vi "15_NOV_UPDATE.vi"() -> ()   [LabVIEW 2020]
uses:
  <vilib>/Utility/file.llb/Write Delimited Spreadsheet (DBL).vi
  <instrlib>/Agilent B2900 Series/Agilent B2900 Series.lvlib
panel:
  in  "Save Data":bool
  out "Y -axis":string
  out "X -axis":string
  out "String":string
  out "SCPI Command":string
  out "?":bool
  in  "Time interval between iterations (seconds)":dbl
  out "?":cluster{"X":dbl[], "Y":dbl[]}[](graph)
  out "Waveform Chart":dbl(graph)
  out "Measured Output Value":dbl
  in  "SELECT DEVICE":refnum<visa-resource-name>="USB0::0x0957::0x8E18::MY51140695::INSTR"
  out "Resolution":dbl format="%#_6f"
  out "Instantaneous Input Value":dbl format="%#_6f"
  in  "Final Value":dbl
  in  "Initial Value":dbl
  in  "Steps":dbl
  in  "Measure (OUTPUT)":enum16{"Voltage", "Current"}(ring)
  in  "Source":enum16{"Voltage", "Current"}(ring)
  in  "Channel":u16(ring) items=["1", "2"]
  # "(INPUT)"
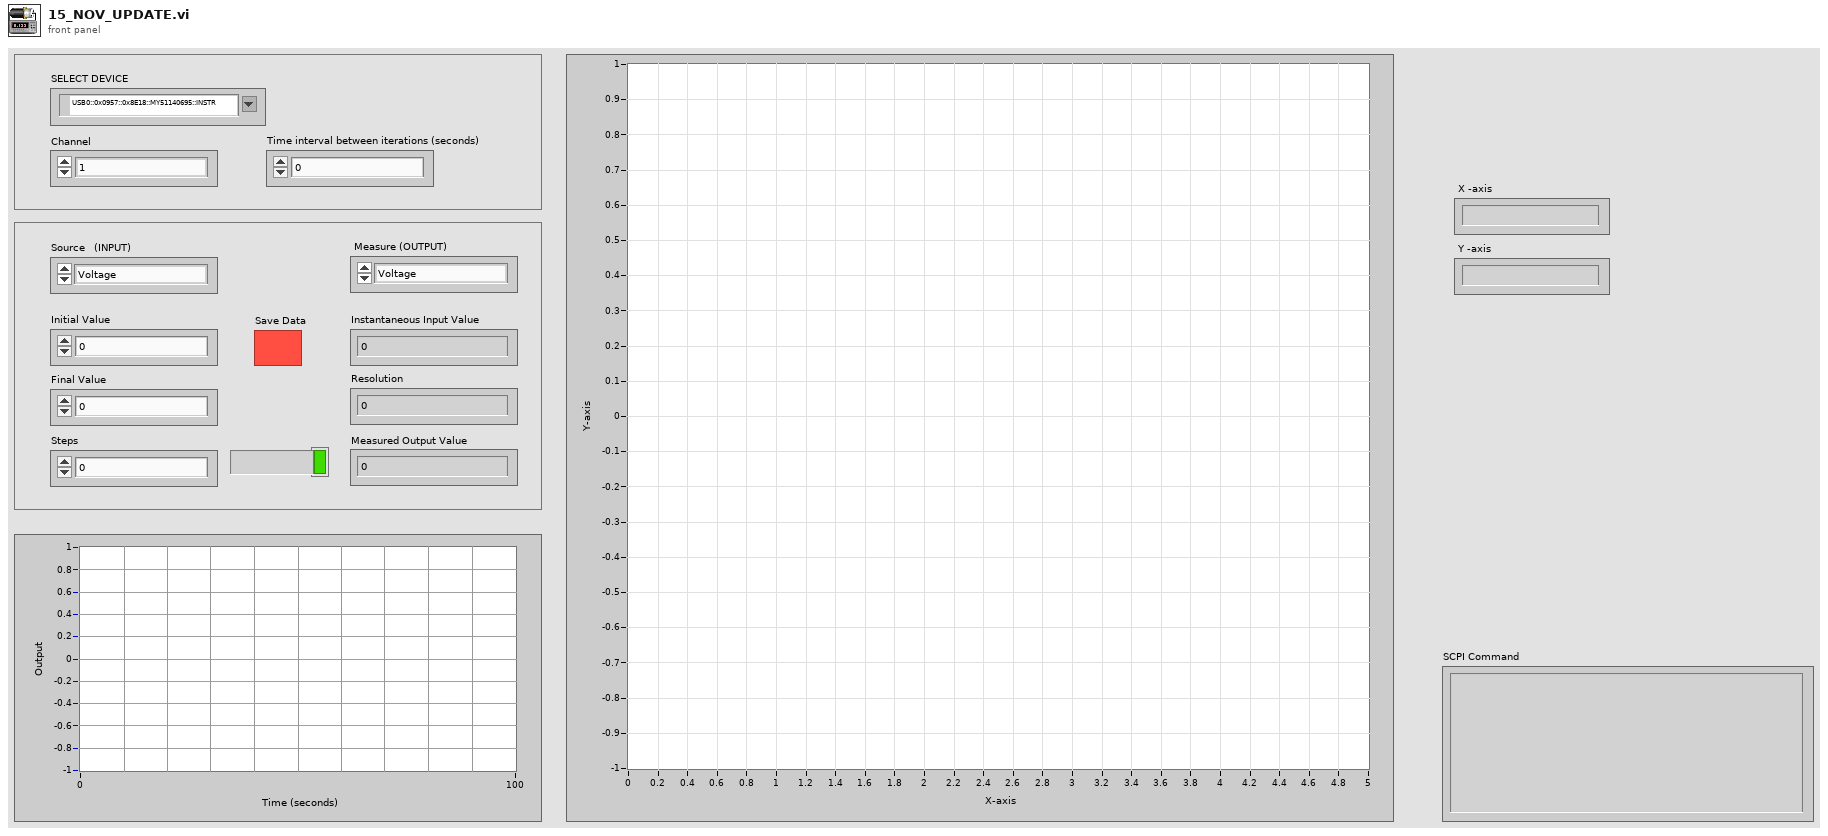
[diagram p1: front panel]
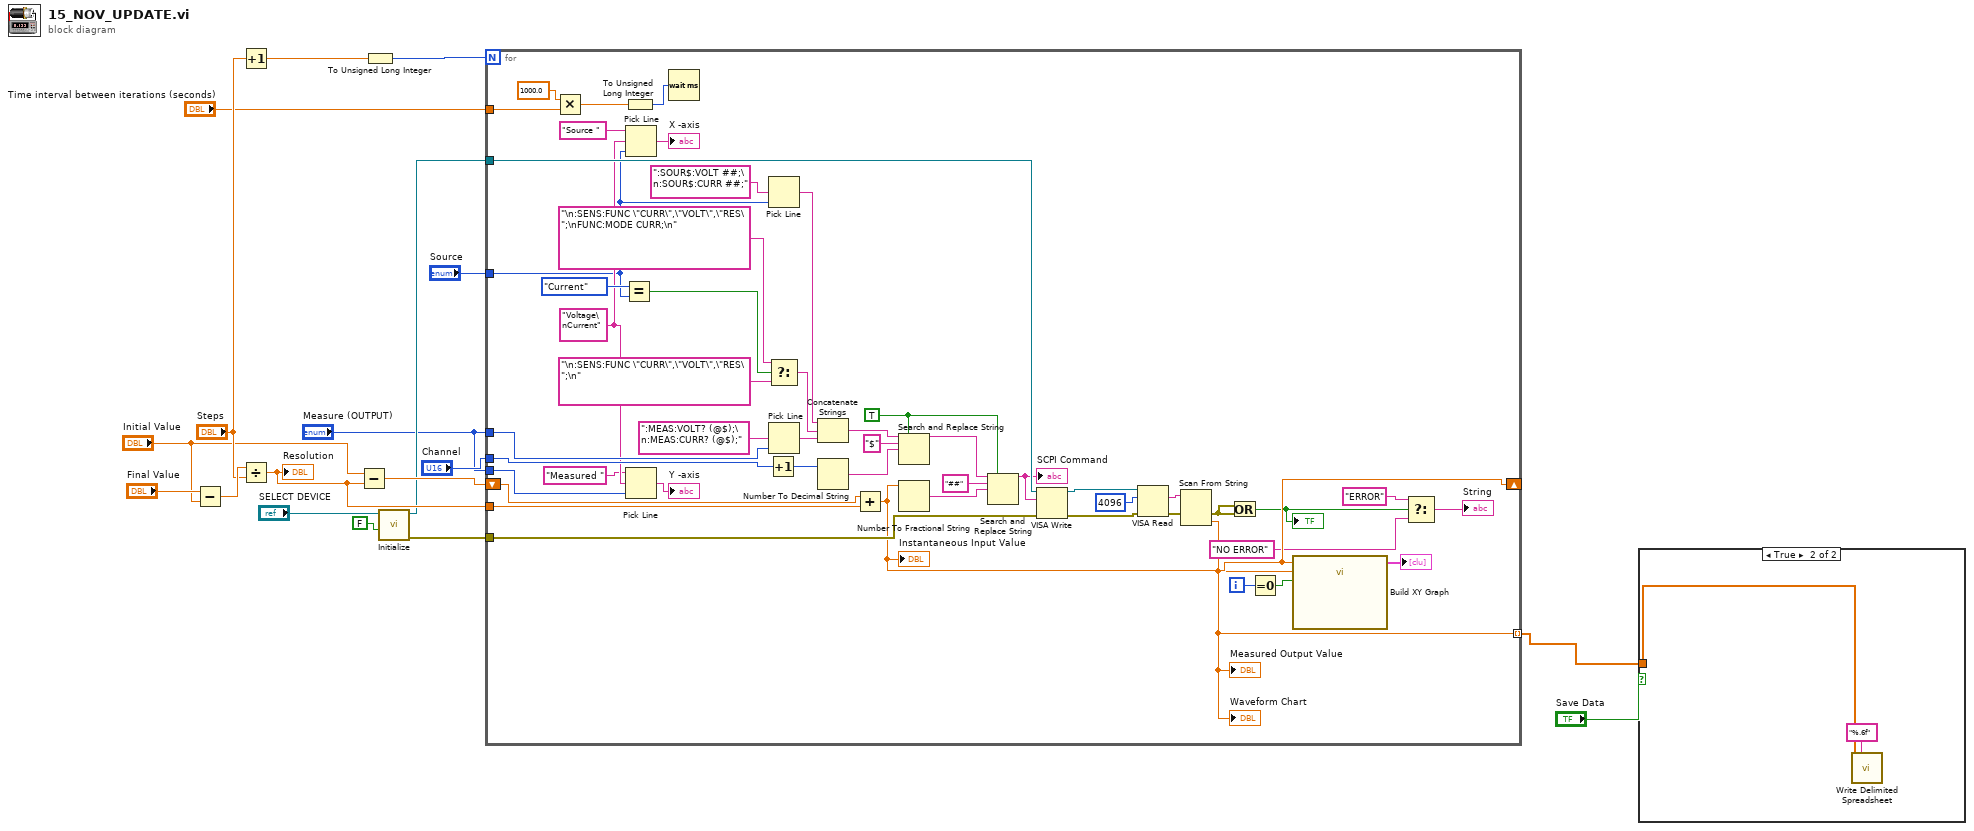
[diagram p0: block diagram]
diagram:
  n1 = Subtract(x="Final Value", y="Initial Value") -> (x-y=w14:dbl)
  n2 = Increment(x="Steps") -> (x+1=w5:dbl)
  n3 = Divide(x=w14, y="Steps") -> (x/y=w13:dbl)
  "Resolution" <- w13
  n4 = Subtract(x="Initial Value", y=w13) -> (x-y=w15:dbl)
  n5 = To Unsigned Long Integer(number=w5) -> (unsigned 32bit integer=w4:u32)
  n6 = call <instrlib>:"Initialize.vi"("Reset (True)"=FALSE, "VISA resource name"="SELECT DEVICE") -> ("error out"=w8:errorcluster, "VISA resource name out"=w9:refnum<visa-resource-name>)  [unwired: 8 in]
  n7 = for {
    N: w4 -> [_]
    tunnel: "Channel" -> [w67]
    tunnel: "Source" -> [w24]
    tunnel: "Measure (OUTPUT)" -> [w65]
    tunnel: w13 -> [w53]
    shift-right: [w41] -> _
    shift-left: w15 -> [w54]
    tunnel: w9 -> [w44]
    tunnel: w8 -> [w43]
    tunnel: "Time interval between iterations (seconds)" -> [w38]
    tunnel: "Measure (OUTPUT)" -> [w23]
    tunnel: [w19] -> w2 mode=indexing
    i -> [w40]
    w25 = "Voltage\nCurrent" ("multi-line string")
    w56 = TRUE ("replace all? (F)")
    n8 = Multiply(x=1000.0, y=w38) -> (x*y=w35:dbl)
    n9 = Equal?(x=enum16{"Voltage", "Current"}."Current", y=w24) -> (x = y?=w50:bool)
    n10 = To Unsigned Long Integer(number=w35) -> (unsigned 32bit integer=w36:u32)
    n11 = Pick Line(string ("")="Source ", multi-line string=w25, line index=w24) -> (output string=→"X -axis":string)
    n12 = Pick Line(string ("")="Measured ", multi-line string=w25, line index=w23) -> (output string=→"Y -axis":string)
    n13 = Wait (ms)(milliseconds to wait=w36) -> ()  [unwired: 1 out]
    n14 = Increment(x=w67) -> (x+1=w60:u16)
    n15 = Pick Line(multi-line string=":SOUR$:VOLT ##;\n:SOUR$:CURR ##;", line index=w24) -> (output string=w63:string)  [unwired: 1 in]
    n16 = Select(t="\n:SENS:FUNC \"CURR\",\"VOLT\",\"RES\";\nFUNC:MODE CURR;\n" ("string"), s=w50, f="\n:SENS:FUNC \"CURR\",\"VOLT\",\"RES\";\n") -> (s? t:f=w48:string)
    n17 = Pick Line(multi-line string=":MEAS:VOLT? (@$);\n:MEAS:CURR? (@$);", line index=w65) -> (output string=w64:string)  [unwired: 1 in]
    n18 = Concatenate Strings(w63, w48, w64) -> (w62:string)
    n19 = Number To Decimal String(number=w60) -> (decimal integer string=w59:string)  [unwired: 1 in]
    n20 = Add(x=w54, y=w53) -> (x+y=w41:dbl)
    "Instantaneous Input Value" <- w41
    n21 = Search and Replace String(replace all?=w56, input string=w62, search string="$", replace string=w59) -> (result string=w58:string)  [unwired: 4 in, 3 out]
    n22 = Number To Fractional String(number=w41) -> (F-format string=w55:string)  [unwired: 3 in]
    n23 = Search and Replace String(replace all?=w56, input string=w58, search string="##", replace string=w55) -> (result string=w33:string)  [unwired: 4 in, 3 out]
    "SCPI Command" <- w33
    n24 = VISA Write(VISA resource name=w44, write buffer=w33, error in (no error)=w43) -> (VISA resource name out=w45:refnum<visa-resource-name>, error out=w46:errorcluster)  [unwired: 1 out]
    n25 = VISA Read(VISA resource name=w45, byte count=u32 4096, error in (no error)=w46) -> (read buffer=w42:string, error out=w32:errorcluster)  [unwired: 2 out]
    n26 = Scan From String(input string=w42, error in=w32) -> (error out=w34:errorcluster, output 1=w19:dbl)  [unwired: 3 in, 2 out]
    "Measured Output Value" <- w19
    "Waveform Chart" <- w19
    n27 = Or(x=w34, y=w34) -> (x .or. y?=w29:bool)
    "?" <- w29
    n28 = Equal To 0?(x=w40) -> (x = 0?=w39:bool)
    n29 = call "Build XY Graph"("Reset"=w39, "Y Input"=w19, "X Input"=w41) -> ("XY Graph"=→"?":cluster{"X":dbl[], "Y":dbl[]}[])  [unwired: 7 in, 1 out]
    n30 = Select(t="ERROR", s=w29, f="NO ERROR") -> (s? t:f=→"String":string)
  }
  n31 = case shown="True" "Save Data" {
    tunnel: w2 -> [_ w70]
    frame False {
    }
    frame True {
      n32 = call-poly <vilib>:"Write Delimited Spreadsheet.vi"("format (%.3f)"="%.6f", "1D data"=w70) -> ()  [unwired: 12 in, 2 out]
    }
  }
